vi "FindCoincidences.vi"(0 "Leftover candidates time":u64, 5 "Primary hits":T1, 7 "Secondary hits":T4(array[cluster]), 11 "Window":i32) -> (4 "Primary hits out":T1, 6 "Secondary hits out":T4(array[cluster]), 8 "Coincidences":T5[](array[typedef]), 10 "Primary hits sorted":T2, 15 "Secondary hits sorted":T3(array[cluster]))   [LabVIEW 2016]
uses:
  Typedefs/Coincidence.ctl
  Global Variables/System info.vi
panel:
  out "Secondary ID":i8
  out "Primary ID":i8
  # "This VI looks for coincidences among five scintillators. One is a primary channel, and four are secondary channels.\nFor each hit on the primary channel, the VI will look for hits on the secondary channels that came within \"window\"\nnanoseconds before or after the primary hit. Each coincidence is put in the \"Coincidences\" array. A clever algorithm makes\nit relativelt fast by not needing to look through the entire secondaries-array before understanding that it will not find a hit\nwithin the specified window.\n\nThe primary hits are sorted based on whether the hit was part of a coincidence or not. This info is put in the \"Primary \nhits sorted\" array. \nThe secondaries are also sorted in this way, but in a way that makes sure that a single hit on a secondary channel can not\nbe counted as being part of two coincidences."
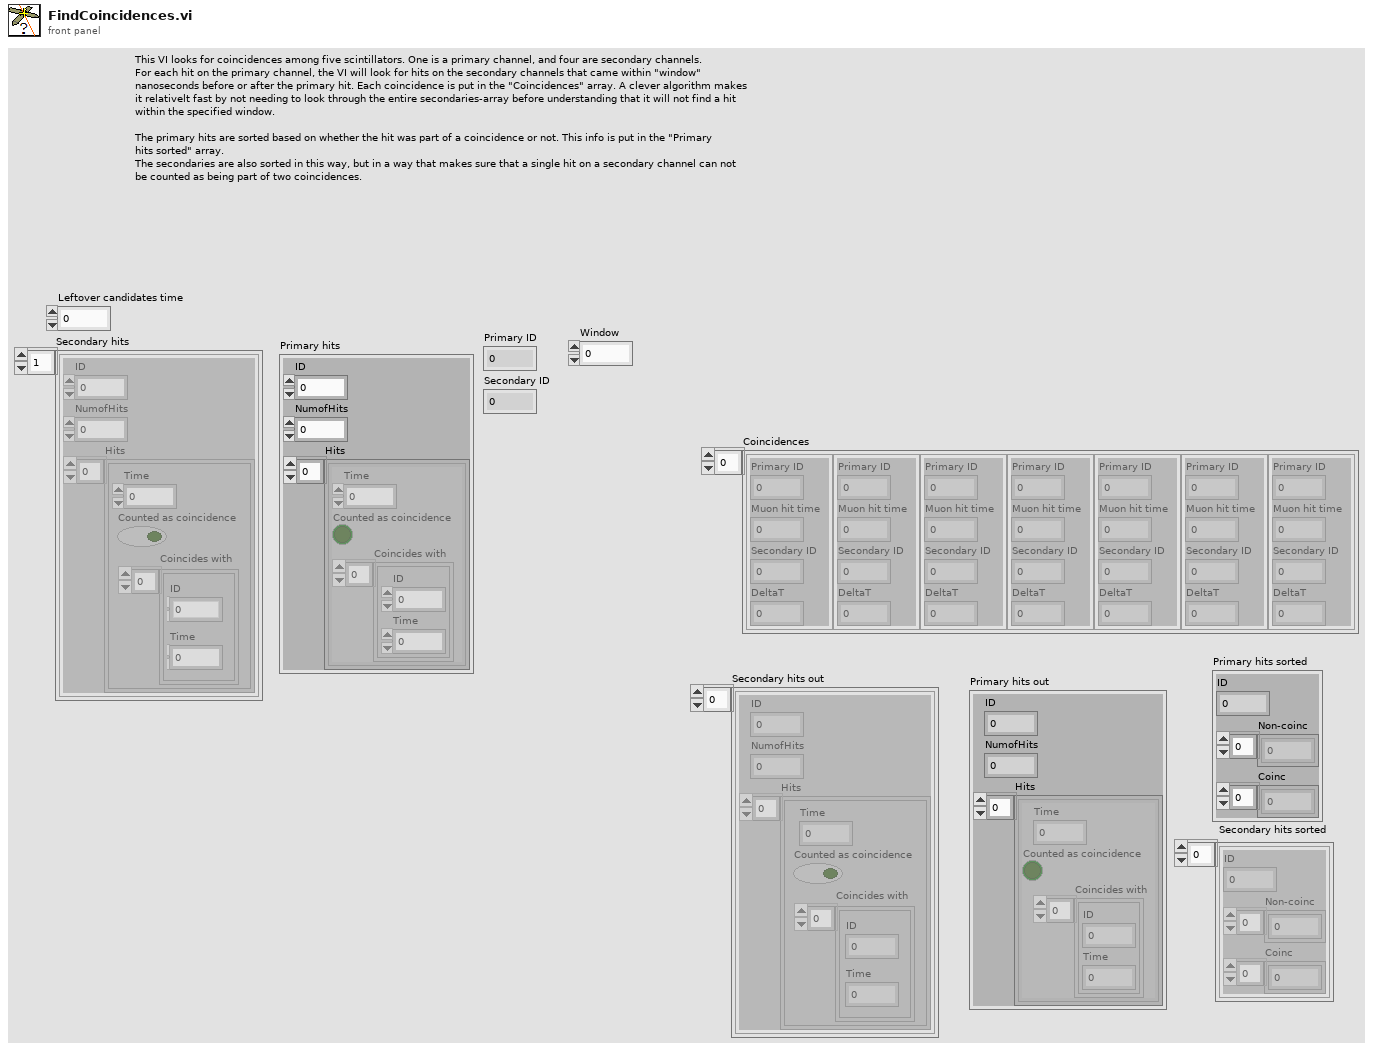
[diagram p1: front panel]
types:
  T1 = cluster{"ID":i8, "NumofHits":i32, "Hits":cluster{"Time":u64, "Counted as coincidence":bool, "Coincides with":cluster{"ID":i8, "Time":u64}[]}[]}
  T2 = cluster{"ID":i8, "Non-coinc":u64[], "Coinc":u64[]}
  T3 = cluster{"ID":i8, "Non-coinc":u64[], "Coinc":u64[]}[]
  T4 = cluster{"ID":i8, "NumofHits":i32, "Hits":cluster{"Time":u64, "Counted as coincidence":bool, "Coincides with":cluster{"ID":i8, "Time":u64}[]}[]}[]
  T5 = typedef "Coincidence.ctl" = cluster{"Primary ID":i8, "Muon hit time":u64, "Secondary ID":i8, "DeltaT":i32}
  T6 = cluster{"Time":u64, "Counted as coincidence":bool, "Coincides with":cluster{"ID":i8, "Time":u64}[]}[]
  T7 = cluster{"Time":u64, "Counted as coincidence":bool, "Coincides with":cluster{"ID":i8, "Time":u64}[]}
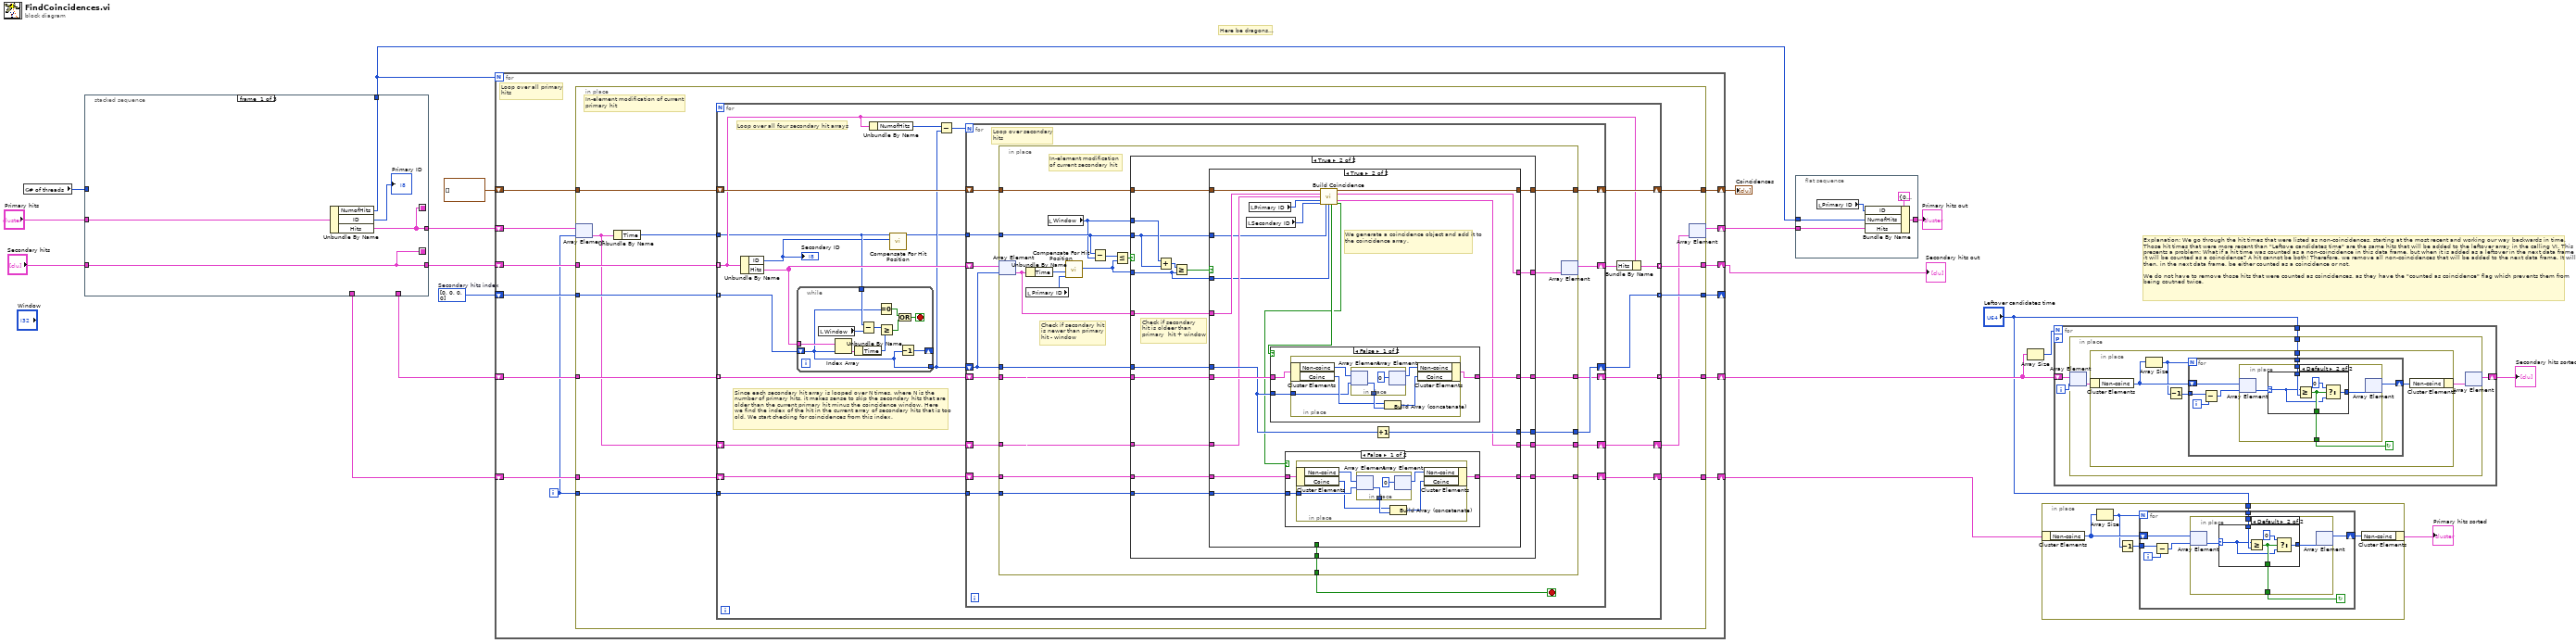
[diagram p0: block diagram]
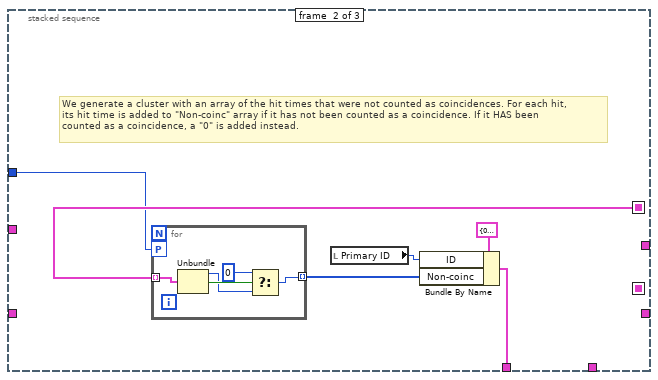
[diagram p2: hidden frame]
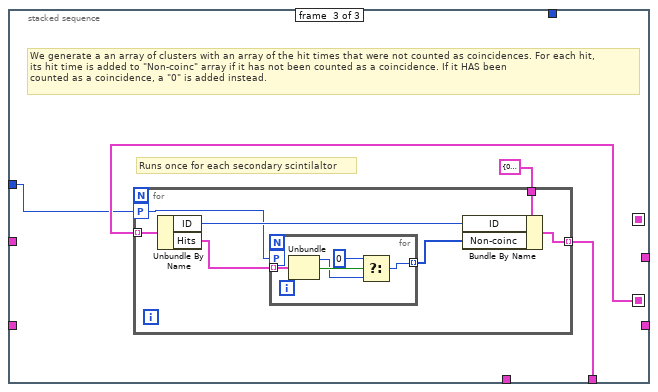
[diagram p3: hidden frame]
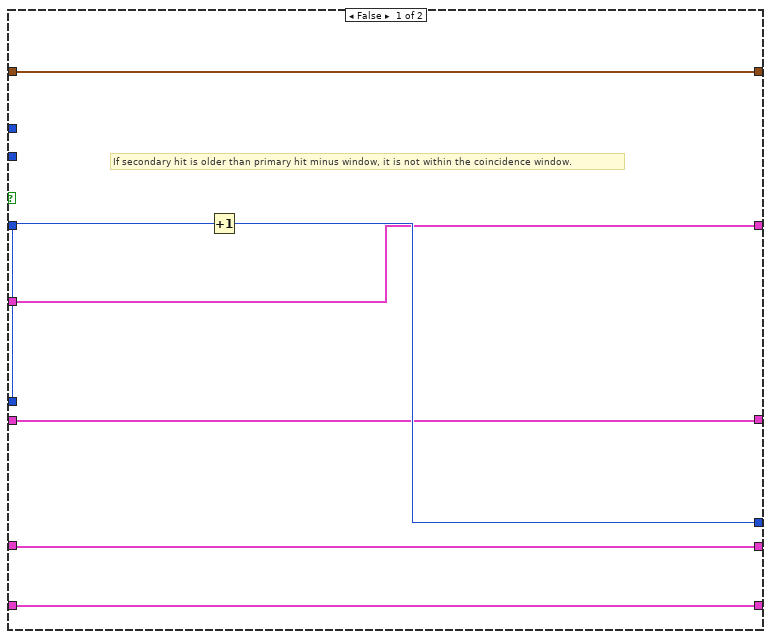
[diagram p6: hidden frame]
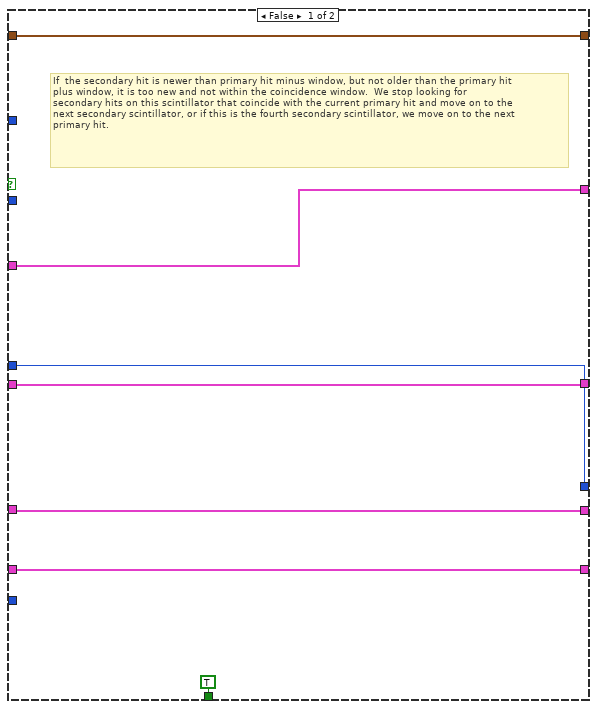
[diagram p7: hidden frame]
diagram:
  w6 = i32[] [0, 0, 0, 0]  # Secondary hits index
  # "Explanation: We go through the hit times that were listed as non-coincidences, starting at the most recent and working our way backwards in time.\nThose hit times that were more recent than \"Leftove candidates time\" are the same hits that will be added to the leftover array in the calling VI. This \npresents a problem: What if a hit time was counted as a non-coincidence in this data frame, but when it is added as a leftover in the next data frame\nit will be counted as a coincidence? A hit cannot be both! Therefore, we remove all non-coincidences that will be added to the next data frame. It will\nthen, in the next data frame, be either counted as a coincidence or not. \n\nWe do not have to remove those hits that were counted as coincidences, as they have the \"counted as coincidence\" flag which prevents them from\nbeing coutned twice."
  # "Here be dragons..."
  n1 = global read "System info.vi" "# of threads"() -> (w1:i32)
  n2 = stacked-sequence {
    seq-local: [w23 _ _] -> [_ w29 _]
    seq-local: [w21 _ _] -> [_ _ w39]
    tunnel: "Secondary hits" -> [w21 _ _]
    tunnel: [w21 _ _] -> w17
    tunnel: [w23 _ _] -> w16
    tunnel: [w25 _ _] -> w3
    tunnel: [_ w28 _] -> w7
    tunnel: [_ _ w38] -> w8
    tunnel: "Primary hits" -> [w22 _ _]
    tunnel: w1 -> [_ w26 w37]
    frame #0 {
      n3 = Unbundle By Name(w22) -> ("NumofHits"=w25:i32, "ID"=→"Primary ID":i8, "Hits"=w23:T6)
    }
    frame #1 {
      # "We generate a cluster with an array of the hit times that were not counted as coincidences. For each hit,\nits hit time is added to \"Non-coinc\" array if it has not been counted as a coincidence. If it HAS been\ncounted as a coincidence, a \"0\" is added instead."
      n4 = for {
        tunnel: w29 -> [w36] mode=indexing
        tunnel: [w32] -> w31 mode=indexing
        workers-P: w26 -> [_]
        n5 = Unbundle(w36) -> ("Time"=w34:u64, "Counted as coincidence"=w35:bool)  [unwired: 1 out]
        n6 = Select(t=u64 0, s=w35, f=w34) -> (s? t:f=w32:u64)
      }
      n7 = local read "Primary ID"() -> (w27:i8)
      n8 = Bundle By Name(cluster=T2 {"ID"=0, "Non-coinc"=[], "Coinc"=[]}, "ID"=w27, "Non-coinc"=w31) -> (w28:T2)
    }
    frame #2 {
      # "Runs once for each secondary scintilaltor"
      # "We generate a an array of clusters with an array of the hit times that were not counted as coincidences. For each hit,\nits hit time is added to \"Non-coinc\" array if it has not been counted as a coincidence. If it HAS been\ncounted as a coincidence, a \"0\" is added instead."
      n9 = for {
        tunnel: w39 -> [w47] mode=indexing
        tunnel: T2 {"ID"=0, "Non-coinc"=[], "Coinc"=[]} -> [w46]
        tunnel: [w44] -> w38 mode=indexing
        workers-P: w37 -> [w41]
        n10 = Unbundle By Name(w47) -> ("ID"=w45:i8, "Hits"=w43:T6)
        n11 = for {
          tunnel: w43 -> [w52] mode=indexing
          tunnel: [w48] -> w42 mode=indexing
          workers-P: w41 -> [_]
          n12 = Unbundle(w52) -> ("Time"=w50:u64, "Counted as coincidence"=w51:bool)  [unwired: 1 out]
          n13 = Select(t=u64 0, s=w51, f=w50) -> (s? t:f=w48:u64)
        }
        n14 = Bundle By Name(cluster=w46, "ID"=w45, "Non-coinc"=w42) -> (w44:T2)
      }
    }
  }
  n15 = for {
    N: w3 -> [_]
    shift-right: [w63] -> w20
    shift-left: T5[] [] -> [w62]
    shift-right: [w61] -> _
    shift-left: w6 -> [w64]
    shift-right: [w59] -> w12
    shift-left: w8 -> [w60]
    shift-right: [w57] -> w10
    shift-left: w7 -> [w58]
    shift-right: [w56] -> w4
    shift-left: w17 -> [w65]
    shift-right: [w53] -> w15
    shift-left: w16 -> [w55]
    i -> [w54]
    # "Loop over all primary\nhits"
    n16 = in-place {
      in-place-border: w65 -> [w79]
      in-place-border: w64 -> [w78]
      in-place-border: [w77] -> w63
      in-place-border: w62 -> [w76]
      in-place-border: [w75] -> w61
      in-place-border: w60 -> [w74]
      in-place-border: [w73] -> w59
      in-place-border: w58 -> [w72]
      in-place-border: [w71] -> w57
      in-place-border: [w70] -> w56
      in-place-border: w54 -> [w69]
      # "In-element modification of current\nprimary hit"
      n17 = in-place-array #1(w55, w54) -> (w66:T7)
      n18 = Unbundle By Name(w66) -> ("Time"=w68:u64)
      n19 = for {
        tunnel: w79 -> [w86] mode=indexing
        tunnel: w78 -> [w97] mode=indexing
        shift-right: [w100] -> w77
        shift-left: w76 -> [w99]
        tunnel: [w98] -> w75 mode=indexing
        tunnel: w74 -> [w96] mode=indexing
        tunnel: [w95] -> w73 mode=indexing
        shift-right: [w93] -> w71
        shift-left: w72 -> [w94]
        tunnel: [w90] -> w70 mode=indexing
        tunnel: w69 -> [w89]
        tunnel: w68 -> [w82]
        shift-right: [w88] -> w67
        shift-left: w66 -> [w87]
        # "Since each secondary hit array is looped over N times, where N is the\nnumber of primary hits, it makes sense to skip the secondary hits that are \nolder than the current primary hit minus the coincidence window. Here \nwe find the index of the hit in the current array of secondary hits that is too \nold. We start checking for coincidences from this index."
        # "Loop over all four secondary hit arrays"
        n20 = Unbundle By Name(w86) -> ("ID"=w81:i8, "Hits"=w92:T6)
        "Secondary ID" <- w81
        n21 = while {
          tunnel: w92 -> [w223]
          tunnel: w82 -> [w222]
          shift-right: [w220] -> _
          shift-left: w97 -> [w219]
          tunnel: [w219] -> w84
          stop <- w216 stop-if-true
          n22 = local read "Window"() -> (w213:i32)
          n23 = Index Array(array=w223, index=w219) -> (element=w215:T7)
          n24 = Unbundle By Name(w215) -> ("Time"=w214:u64)
          n25 = Subtract(x=w222, y=w213) -> (x-y=w221:u64)
          n26 = Equal To 0?(x=w219) -> (x = 0?=w217:bool)
          n27 = Greater Or Equal?(x=w221, y=w214) -> (x >= y?=w218:bool)
          n28 = Or(x=w217, y=w218) -> (x .or. y?=w216:bool)
          n29 = Decrement(x=w219) -> (x-1=w220:i32)
        }
        n30 = Unbundle By Name(w86) -> ("NumofHits"=w85:i32)
        n31 = call "Compensate For Hit Position.vi"("Secondary channel"=w81, "Primary hit time"=w82) -> ("Primary true hit time"=w80:u64)  [unwired: 8 in, 1 out]
        n32 = Subtract(x=w85, y=w84) -> (x-y=w83:i32)
        n33 = for {
          N: w83 -> [_]
          tunnel: w80 -> [w113]
          shift-right: [w114] -> w98
          shift-left: w84 -> [w110]
          shift-right: [w112] -> w100
          shift-left: w99 -> [w111]
          shift-right: [w104] -> w95
          shift-left: w96 -> [w109]
          shift-right: [w105] -> w93
          shift-left: w94 -> [w108]
          shift-right: [w107] -> w91
          shift-left: w92 -> [w115]
          tunnel: w89 -> [w106]
          shift-right: [w103] -> w88
          shift-left: w87 -> [w102]
          stop <- w101 stop-if-true
          # "Loop over secondary\nhits"
          n34 = in-place {
            in-place-border: [w134] -> w114
            in-place-border: w113 -> [w133]
            in-place-border: [w132] -> w101
            in-place-border: [w131] -> w112
            in-place-border: w111 -> [w130]
            in-place-border: w110 -> [w129]
            in-place-border: w108 -> [w126]
            in-place-border: w106 -> [w124]
            in-place-border: w109 -> [w125]
            in-place-border: [w123] -> w105
            in-place-border: [w122] -> w104
            in-place-border: w102 -> [w121]
            in-place-border: [w120] -> w103
            # "Check if secondary hit\nis newer than primary \nhit - window"
            # "In-element modification \nof current secondary hit"
            n35 = in-place-array #2(w115, w110) -> (w127:T7)
            n36 = Unbundle By Name(w127) -> ("Time"=w118:u64)
            n37 = local read "Primary ID"() -> (w117:i8)
            n38 = local read "Window"() -> (w119:i32)
            n39 = call "Compensate For Hit Position.vi"("Primary channel"=w117, "Secondary hit time"=w118) -> ("Secondary true hit time"=w116:u64)  [unwired: 8 in, 1 out]
            n40 = Subtract(x=w133, y=w119) -> (x-y=w136:u64)
            n41 = Less Or Equal?(x=w136, y=w116) -> (x <= y?=w135:bool)
            n42 = case shown="True" w135 {
              tunnel: w129 -> [w143 w160]
              tunnel: [w142 w159] -> w134
              tunnel: w133 -> [_ w145]
              tunnel: w116 -> [_ w144]
              tunnel: [_ w158] -> w132
              tunnel: [w141 w157] -> w131
              tunnel: w130 -> [w141 w156]
              tunnel: w127 -> [w140 w155]
              tunnel: [w140 w154] -> w128
              tunnel: w126 -> [w138 w153]
              tunnel: w125 -> [w139 w152]
              tunnel: w124 -> [_ w151]
              tunnel: [w138 w150] -> w123
              tunnel: [w139 w149] -> w122
              tunnel: w121 -> [w137 w148]
              tunnel: [w137 w147] -> w120
              tunnel: w119 -> [_ w146]
              frame False {
                # "If secondary hit is older than primary hit minus window, it is not within the coincidence window."
                n43 = Increment(x=w143) -> (x+1=w142:i32)
              }
              frame True {
                # "Check if secondary \nhit is oldeer than \nprimary  hit + window"
                n44 = Add(x=w146, y=w145) -> (x+y=w162:u64)
                n45 = Greater Or Equal?(x=w162, y=w144) -> (x >= y?=w161:bool)
                n46 = case shown="True" w161 {
                  tunnel: w160 -> [w169 w183]
                  tunnel: [w169 w188] -> w159
                  tunnel: [TRUE _] -> w158
                  tunnel: [w167 w187] -> w157
                  tunnel: w156 -> [w167 w178]
                  tunnel: w155 -> [w166 w177]
                  tunnel: [w166 w175] -> w154
                  tunnel: w153 -> [w165 w186]
                  tunnel: w152 -> [w164 w184]
                  tunnel: w151 -> [_ w185]
                  tunnel: [w165 w182] -> w150
                  tunnel: [w164 w181] -> w149
                  tunnel: w148 -> [w163 w176]
                  tunnel: [w163 w174] -> w147
                  tunnel: w145 -> [_ w171]
                  tunnel: w144 -> [_ w170]
                  frame False {
                    # "If  the secondary hit is newer than primary hit minus window, but not older than the primary hit \nplus window, it is too new and not within the coincidence window.  We stop looking for \nsecondary hits on this scintillator that coincide with the current primary hit and move on to the\nnext secondary scintillator, or if this is the fourth secondary scintillator, we move on to the next\nprimary hit."
                  }
                  frame True {
                    # "We generate a coincidence object and add it to the coincidence array."
                    n47 = local read "Secondary ID"() -> (w179:i8)
                    n48 = local read "Primary ID"() -> (w180:i8)
                    n49 = call "Build Coincidence.vi"("Coincs in"=w178, "Secondary hit in"=w177, "Primary hit in"=w176, "Primary ID"=w180, "Secondary ID"=w179, "Primary true hit time"=w171, "Secondary true hit time"=w170) -> ("Coincs out"=w187:T5[], "Secondary hit out"=w175:T7, "Primary hit out"=w174:T7, "secondary counted as coinc"=w173:bool, "Primary counted as coinc"=w172:bool)  [unwired: 4 in]
                    n50 = case shown="False" w173 {
                      tunnel: w184 -> [w191 w200]
                      tunnel: w183 -> [w190 _]
                      tunnel: [w189 w200] -> w181
                      frame False {
                        n51 = in-place {
                          in-place-border: w190 -> [w192]
                          n52 = in-place-cluster #3(w191) -> ("Non-coinc"=w197:u64[], "Coinc"=w194:u64[])
                          n53 = in-place {
                            in-place-border: [w198] -> w195
                            n54 = in-place-array #4(w197, w192) -> (w198:u64)
                            n55 = in-place-array #4(u64 0 ("element")) -> (w196:u64[])  [unwired: 1 out]
                          }
                          n56 = Build Array (concatenate)(w194, w195) -> (w193:u64[])
                          n57 = in-place-cluster #3("Non-coinc"=w196, "Coinc"=w193) -> (w189:T2)
                        }
                      }
                      frame True {
                      }
                    }
                    n58 = case shown="False" w172 {
                      tunnel: [w201 w212] -> w182
                      tunnel: w186 -> [w203 w212]
                      tunnel: w185 -> [w202 _]
                      frame False {
                        n59 = in-place {
                          in-place-border: w202 -> [w208]
                          n60 = in-place-cluster #5(w203) -> ("Non-coinc"=w209:u64[], "Coinc"=w205:u64[])
                          n61 = in-place {
                            in-place-border: [w210] -> w206
                            n62 = in-place-array #6(w209, w208) -> (w210:u64)
                            n63 = in-place-array #6(u64 0 ("element")) -> (w207:u64[])  [unwired: 1 out]
                          }
                          n64 = Build Array (concatenate)(w205, w206) -> (w204:u64[])
                          n65 = in-place-cluster #5("Non-coinc"=w207, "Coinc"=w204) -> (w201:T2)
                        }
                      }
                      frame True {
                      }
                    }
                    n66 = Increment(x=w183) -> (x+1=w188:i32)
                  }
                }
              }
            }
            n67 = in-place-array #2(w128) -> (w107:T6)  [unwired: 1 out]
          }
        }
        n68 = Bundle By Name(cluster=w86, "Hits"=w91) -> (w90:T1)
      }
      n69 = in-place-array #1(w67) -> (w53:T6)  [unwired: 1 out]
    }
  }
  "Coincidences" <- w20
  "Secondary hits out" <- w4
  n70 = flat-sequence {
    tunnel: w15 -> [w228]
    tunnel: w3 -> [w226]
    tunnel: [w224] -> w2
    frame #0 {
      n71 = local read "Primary ID"() -> (w225:i8)
      n72 = Bundle By Name(cluster=T1 {"ID"=0, "NumofHits"=0, "Hits"=[]} ("Primary hits"), "ID"=w225, "NumofHits"=w226, "Hits"=w228) -> (w224:T1)
    }
  }
  n73 = Array Size(array=w12) -> (size(s)=w13:i32)
  n74 = in-place {
    in-place-border: "Leftover candidates time" -> [w233]
    n75 = in-place-cluster #7(w10) -> ("Non-coinc"=w232:u64[])
    n76 = Array Size(array=w232) -> (size(s)=w230:i32)
    n77 = Decrement(x=w230) -> (x-1=w231:i32)
    n78 = for {
      N: w230 -> [_]
      tunnel: w233 -> [w239]
      tunnel: w231 -> [w238]
      shift-right: [w235] -> w229
      shift-left: w232 -> [w240]
      i -> [w237]
      stop <- w234 continue-if-true
      n79 = Subtract(x=w238, y=w237) -> (x-y=w236:i32)
      n80 = in-place {
        in-place-border: w239 -> [w244]
        in-place-border: [w242] -> w234
        n81 = in-place-array #8(w240, w236) -> (w241:u64)
        n82 = case shown="Default" w241 {
          selector: w241 -> [w245 w246]
          tunnel: w244 -> [_ w250]
          tunnel: [w245 w248] -> w243
          tunnel: [_ w247] -> w242
          frame 0 {
          }
          frame Default {
            n83 = Greater Or Equal?(x=w246, y=w250) -> (x >= y?=w247:bool)
            n84 = Select(t=u64 0, s=w247, f=w246) -> (s? t:f=w248:u64)
          }
        }
        n85 = in-place-array #8(w243) -> (w235:u64[])  [unwired: 1 out]
      }
    }
    n86 = in-place-cluster #7("Non-coinc"=w229) -> (→"Primary hits sorted":T2)
  }
  n87 = for {
    N: w13 -> [_]
    tunnel: "Leftover candidates time" -> [w252]
    shift-right: [w251] -> w14
    shift-left: w12 -> [w254]
    workers-P: _ -> [_]
    i -> [w253]
    n88 = in-place {
      in-place-border: w252 -> [w256]
      n89 = in-place-array #9(w254, w253) -> (w257:T2)
      n90 = in-place {
        in-place-border: w256 -> [w262]
        n91 = in-place-cluster #10(w257) -> ("Non-coinc"=w261:u64[])
        n92 = Array Size(array=w261) -> (size(s)=w259:i32)
        n93 = Decrement(x=w259) -> (x-1=w260:i32)
        n94 = for {
          N: w259 -> [_]
          tunnel: w262 -> [w268]
          tunnel: w260 -> [w267]
          shift-right: [w264] -> w258
          shift-left: w261 -> [w269]
          i -> [w266]
          stop <- w263 continue-if-true
          n95 = Subtract(x=w267, y=w266) -> (x-y=w265:i32)
          n96 = in-place {
            in-place-border: w268 -> [w273]
            in-place-border: [w271] -> w263
            n97 = in-place-array #11(w269, w265) -> (w270:u64)
            n98 = case shown="Default" w270 {
              selector: w270 -> [w274 w275]
              tunnel: w273 -> [_ w279]
              tunnel: [w274 w277] -> w272
              tunnel: [_ w276] -> w271
              frame 0 {
              }
              frame Default {
                n99 = Greater Or Equal?(x=w275, y=w279) -> (x >= y?=w276:bool)
                n100 = Select(t=u64 0, s=w276, f=w275) -> (s? t:f=w277:u64)
              }
            }
            n101 = in-place-array #11(w272) -> (w264:u64[])  [unwired: 1 out]
          }
        }
        n102 = in-place-cluster #10("Non-coinc"=w258) -> (w255:T2)
      }
      n103 = in-place-array #9(w255) -> (w251:T3)  [unwired: 1 out]
    }
  }
  "Secondary hits sorted" <- w14
  "Primary hits out" <- w2
